vi "REM IO - Get ECAT IOVar Data.vi"(5 "Section Name":string, 6 "VS Refs In":T4 {"Output VS Refs" format="%.0x"; "Input VS Refs" format="%.0x"}, 7 "ECAT Variablenobjekt":refnum<k21>[](array[refnum]), 8 "error in (no error)":errorcluster caption="Fehler (Eingang, kein Fehler)", 9 "I/O Output Vars In":T1[](array[typedef]) {"VS ref" format="%.0x"}, 10 "I/O Input Vars In":T1[](array[typedef]) {"VS ref" format="%.0x"}, 11 "VS ref":T2=18446744073709551615 format="%.0x") -> (0 "error out (Ausgang)":errorcluster caption="Fehler (Ausgang)", 1 "I/O Output Vars Out":T1[](array[typedef]) {"VS ref" format="%.0x"}, 2 "I/O Input Vars Out":T1[](array[typedef]) {"VS ref" format="%.0x"}, 3 "VS ref 2":T2=18446744073709551615 format="%.0x", 4 "VS Refs Out":T4 {"Output VS Refs" format="%.0x"; "Input VS Refs" format="%.0x"})   [LabVIEW 2019, in "SEECD Engine.lvlib"]
uses:
  SEECD Engine.lvlib
  Type Defs/REM IO ECAT Slave IOV Cluster.ctl
  <vilib>/NI VeriStand/Custom Device API/Custom Device Item Ref.ctl
  Shared/Type Defs/UDV Data Type.ctl
  <vilib>/NI VeriStand/Custom Device API/Custom Device Channel Type.ctl
  Shared/SEECD Shared.lvlib
  <resource>/objmgr/ni.var.rc
  <vilib>/NI VeriStand/Custom Device API/Custom Device API.lvlib
  <vilib>/NI VeriStand/Custom Device Tools/Custom Device Utility Library/Custom Device Utility Library.lvlib
panel:
  out "ECAT Variablenobjekt out":refnum<k21>[](array[refnum])
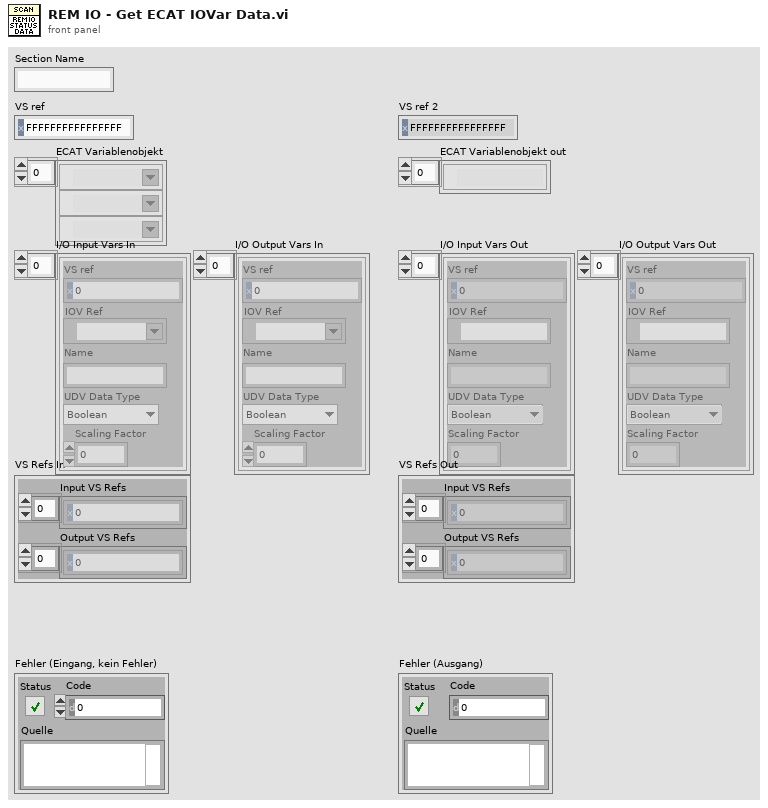
[diagram p1: front panel]
types:
  T1 = typedef "SEECD Engine.lvlib/REM IO ECAT Slave IOV Cluster.ctl" = cluster{"VS ref":T2, "IOV Ref":refnum<k21>, "Name":string, "UDV Data Type":T3, "Scaling Factor":dbl}
  T2 = typedef "Custom Device API.lvlib/Custom Device Item Ref.ctl" = u64
  T3 = typedef "SEECD Shared.lvlib/UDV Data Type.ctl" = enum16{"Boolean", "Fixed Point", "Int8", "Int16", "Int32", "Int64", "U32 Bit Field", "UInt8", "UInt16", "UInt32", "UInt64", "Other", "DBL", "SGL"}
  T4 = cluster{"Input VS Refs":T2[], "Output VS Refs":T2[]}
  T5 = typedef "Custom Device API.lvlib/Custom Device Channel Type.ctl" = enum16{"Input", "Output"}
  T6 = typedef "SEECD Shared.lvlib/ECAT Channel Data Type.ctl" = enum16{"Boolean", "Fixed Point", "Int8", "Int16", "Int32", "Int64", "U32 Bit Field", "UInt8", "UInt16", "UInt32", "UInt64", "Other", "DBL", "SGL"}
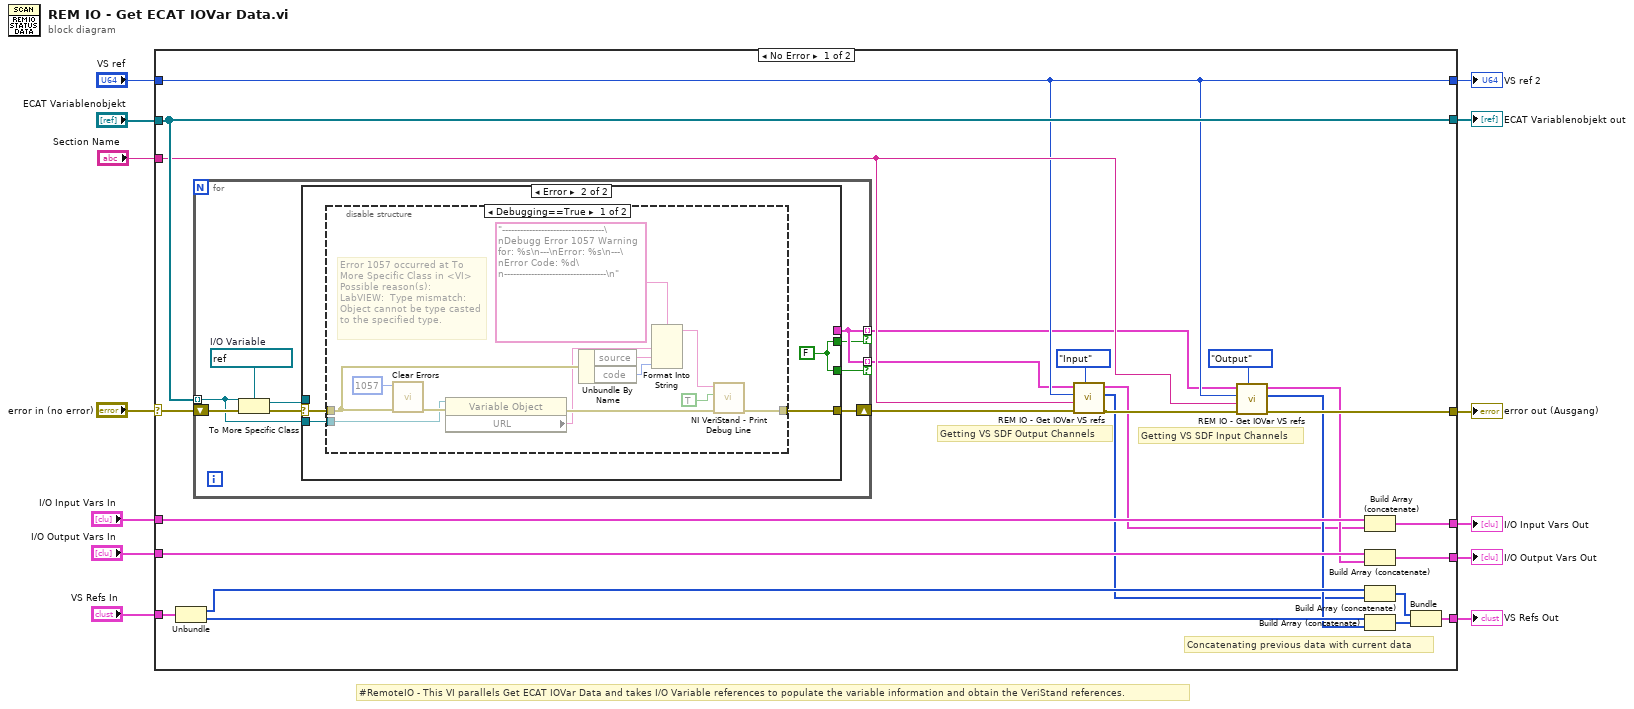
[diagram p0: block diagram]
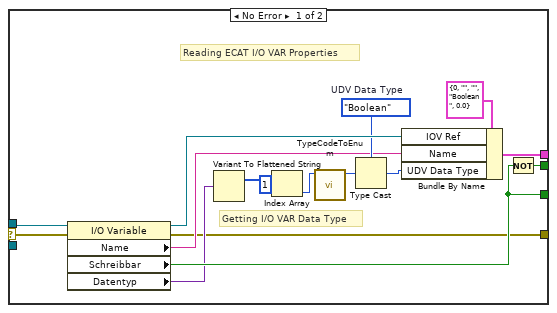
[diagram p2: hidden frame]
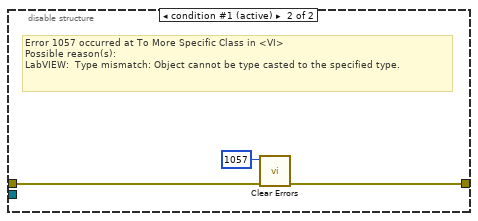
[diagram p3: hidden frame]
diagram:
  # "#RemoteIO - This VI parallels Get ECAT IOVar Data and takes I/O Variable references to populate the variable information and obtain the VeriStand references."
  n1 = case shown="No Error" "error in (no error)" {
    selector: "error in (no error)" -> [w37 w85]
    tunnel: "ECAT Variablenobjekt" -> [w38 w84]
    tunnel: [w21 w85] -> w11
    tunnel: [w38 w84] -> w10
    tunnel: "VS ref" -> [w22 w83]
    tunnel: [w22 w83] -> w8
    tunnel: "Section Name" -> [w23 _]
    tunnel: "VS Refs In" -> [w36 _]
    tunnel: [w31 _] -> w5
    tunnel: "I/O Output Vars In" -> [w30 _]
    tunnel: "I/O Input Vars In" -> [w29 _]
    tunnel: [w28 _] -> w2
    tunnel: [w27 _] -> w1
    frame No Error {
      # "Concatenating previous data with current data"
      # "Getting VS SDF Input Channels"
      # "Getting VS SDF Output Channels"
      n2 = Unbundle(w36) -> ("Input VS Refs"=w34:T2[], "Output VS Refs"=w35:T2[])
      n3 = for {
        shift-right: [w42] -> w26
        shift-left: w37 -> [w41]
        tunnel: w38 -> [w39] mode=indexing
        tunnel: [w47] -> w14 mode=indexing if=w46
        tunnel: [w47] -> w15 mode=indexing if=w45
        w44 = refnum<k21> refnum  # I/O Variable
        n4 = To More Specific Class(target class=w44, reference=w39, error in=w41) -> (specific class reference=w43:refnum<k21>, error out=w40:errorcluster)
        n5 = case shown="Error" w40 {
          selector: w40 -> [w49 w66]
          tunnel: [w62 _] -> w47
          tunnel: [w61 w67] -> w46
          tunnel: [w60 w67] -> w45
          tunnel: w43 -> [w59 _]
          tunnel: [w50 w65] -> w42
          tunnel: w39 -> [_ w64]
          frame No Error {
            w54 = UDV_Data_Type."Boolean"  # UDV Data Type
            # "Reading ECAT I/O VAR Properties"
            # "Getting I/O VAR Data Type"
            n6 = property class="I/O Variable"(reference=w59, error in=w49) -> (reference out=w63:refnum<k21>, error out=w50:errorcluster, "Name"=w52:string, "Schreibbar"=w60:bool, "Datentyp"=w56:variant)
            n7 = Variant To Flattened String(Variant=w56) -> (1:w57:i16[])  [unwired: 1 out]
            n8 = Index Array(array=w57, index=1) -> (element=w55:i16)
            n9 = call "TypeCodeToEnum.vi"("Type Code (numbers in hexadecimal)"=w55) -> ("UDV Data Type"=w53:T6)  [unwired: 9 in, 1 out]
            n10 = Type Cast(type=w54, x=w53) -> (*(type *) &x=w51:T3)
            n11 = Bundle By Name(cluster=T1 {"VS ref"=0, "IOV Ref"="", "Name"="", "UDV Data Type"=enum."Boolean", "Scaling Factor"=0.0} ("ECAT I/O Variable Data"), "IOV Ref"=w63, "Name"=w52, "UDV Data Type"=w51) -> (w62:T1)
            n12 = Not(x=w60) -> (.not. x?=w61:bool)
          }
          frame Error {
            w67 = FALSE
            n13 = disable-structure shown="Debugging==True" {
              disable-tunnel: w66 -> [w77 w81]
              disable-tunnel: [w74 w80] -> w65
              disable-tunnel: w64 -> [w73 _]
              frame condition #0 {
                # "Error 1057 occurred at To More Specific Class in <VI>\nPossible reason(s):\nLabVIEW:  Type mismatch: Object cannot be type casted to the specified type."
                n14 = call <vilib>:"Clear Errors.vi"("error in (no error)"=w77, "specific error code to clear (0: all)"=1057) -> ("error out"=w76:errorcluster)  [unwired: 4 in, 1 out]
                n15 = property class="Variable Object"(reference=w73, error in=w76) -> (error out=w75:errorcluster, "URL"=w72:string)  [unwired: 1 out]
                n16 = Unbundle By Name(w77) -> ("source"=w71:string, "code"=w70:i32)
                n17 = Format Into String(format string="----------------------------------\nDebugg Error 1057 Warning for: %s\n---\nError: %s\n---\nError Code: %d\n----------------------------------\n" ("Format-String"), w72, w71, w70) -> (resulting string=w78:string)  [unwired: 2 in, 1 out]
                n18 = call <vilib>:"NI VeriStand - Print Debug Line.vi"("error in (no error)"=w75, "Add to log file? (F)"=TRUE, "Message"=w78) -> ("error out"=w74:errorcluster)  [unwired: 8 in]
              }
              frame condition #1 (active) {
                # "Error 1057 occurred at To More Specific Class in <VI>\nPossible reason(s):\nLabVIEW:  Type mismatch: Object cannot be type casted to the specified type."
                n19 = call <vilib>:"Clear Errors.vi"("error in (no error)"=w81, "specific error code to clear (0: all)"=1057) -> ("error out"=w80:errorcluster)  [unwired: 4 in, 1 out]
              }
            }
          }
        }
      }
      n20 = call "REM IO - Get IOVar VS refs.vi"("Channel Type"=Custom_Device_Channel_Type."Input", "Fehler (Eingang, kein Fehler)"=w26, "Section Name"=w23, "Item Ref"=w22, "I/O Variable Data in"=w15) -> ("Fehler (Ausgang)"=w24:errorcluster, "Channel Refs"=w18:T2[], "I/O Variable Data out"=w16:T1[])  [unwired: 4 in]
      n21 = call "REM IO - Get IOVar VS refs.vi"("Channel Type"=Custom_Device_Channel_Type."Output", "Fehler (Eingang, kein Fehler)"=w24, "Section Name"=w23, "Item Ref"=w22, "I/O Variable Data in"=w14) -> ("Fehler (Ausgang)"=w21:errorcluster, "Channel Refs"=w19:T2[], "I/O Variable Data out"=w17:T1[])  [unwired: 4 in]
      n22 = Build Array (concatenate)(w29, w16) -> (w28:T1[])
      n23 = Build Array (concatenate)(w30, w17) -> (w27:T1[])
      n24 = Build Array (concatenate)(w34, w18) -> (w32:T2[])
      n25 = Build Array (concatenate)(w35, w19) -> (w33:T2[])
      n26 = Bundle(w32, w33) -> (w31:cluster{T2[], T2[]})  [unwired: 1 in]
    }
    frame Error {
    }
  }
  "I/O Input Vars Out" <- w2
  "I/O Output Vars Out" <- w1
  "error out (Ausgang)" <- w11
  "ECAT Variablenobjekt out" <- w10
  "VS ref 2" <- w8
  "VS Refs Out" <- w5
